vi "PSRR.vi"(11 "数组":dbl[](array[numeric])) -> (2 "PSRR":dbl=122.60591675460435)   [LabVIEW 2019]
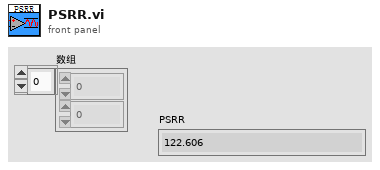
[diagram p1: front panel]
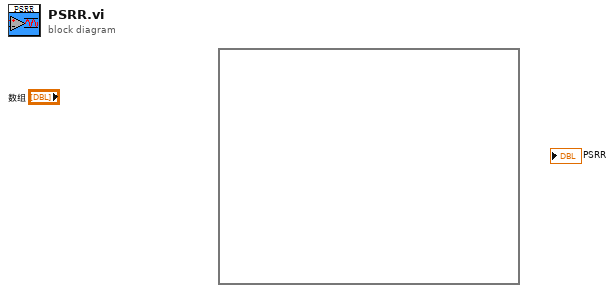
[diagram p0: block diagram]
diagram:
  n1 = formula code=""() -> ()
